vi "Netburner_cntl5.vi"() -> ()   [LabVIEW 2013]
uses:
  <vilib>/Analysis/NI_AALBase.lvlib
panel:
  out "Min ADC":dbl format="%#_5g"
  out "Max ADC":dbl format="%#_5g"
  out "ADC Voltage Chart":dbl(graph)
  out "# Cycles":i32
  out "ADC Std Dev":dbl format="%#_4g"
  out "Mean ADC":dbl format="%#_5g"
  out "ADC error":dbl[](array[numeric])
  out "ADC value":dbl[](array[numeric])
  out "#  Bytes Read End":u32
  out "End string":string
  out "ADC result string":string
  out "#  Bytes Read Data":u32
  in  "DAC, ADC String":string="0 1. 1 -1. 0 100 100"
  out "Error Out":errorcluster={"status"=FALSE, "code"=1073676294, "source"="VISA Read in Netburner_RD.vi->Netburner_cntl.vi"}
  in  "Error In (none)":errorcluster
  in  "COM Port #":refnum<visa-resource-name>="COM3"
  # "Netburner ADC/DAC Test Interface"
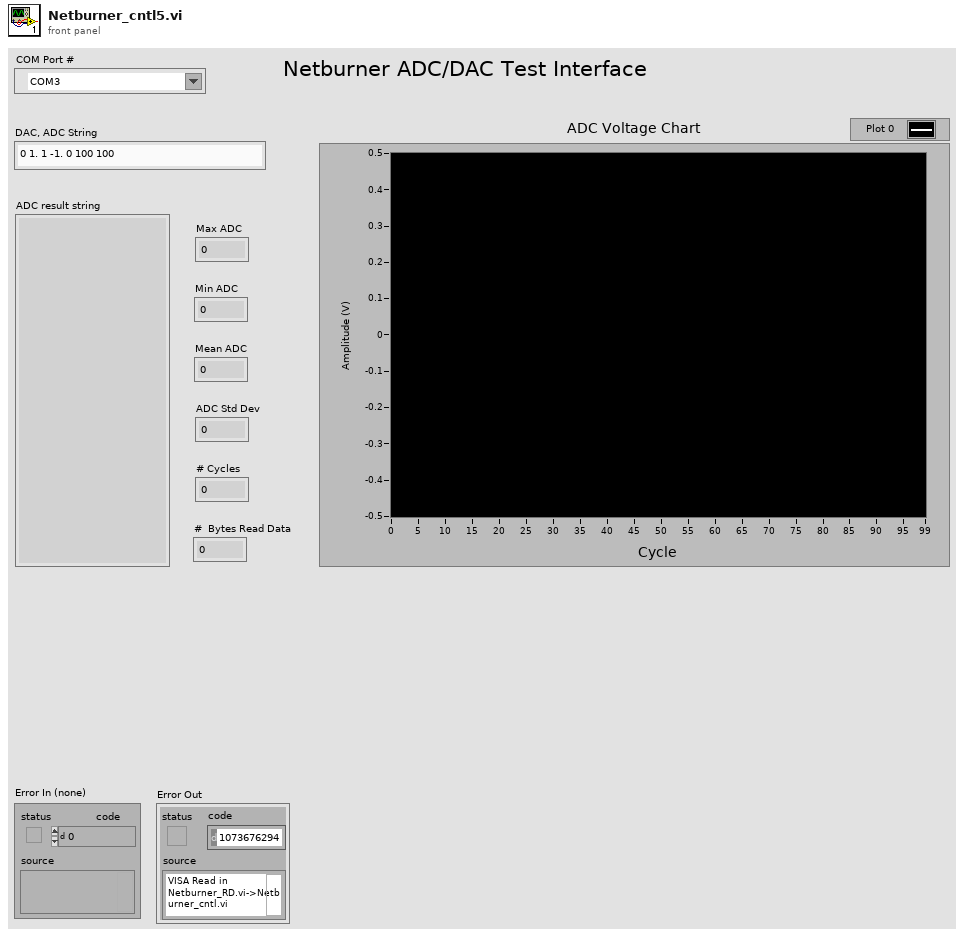
[diagram p1: front panel]
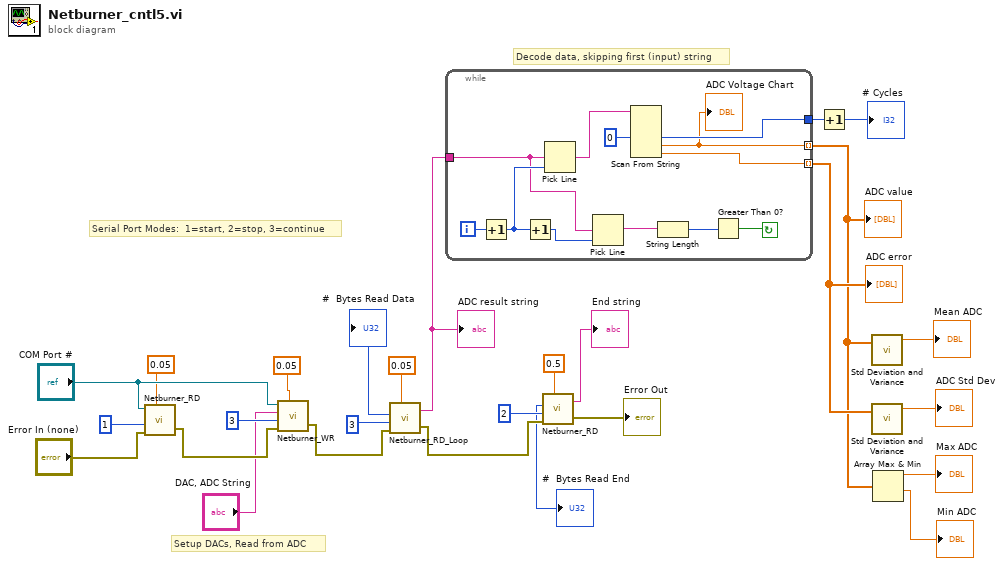
[diagram p0: block diagram]
diagram:
  # "Decode data, skipping first (input) string"
  # "Serial Port Modes:  1=start, 2=stop, 3=continue"
  # "Setup DACs, Read from ADC"
  n1 = call "Netburner_RD.vi"("VISA resource name (COM Port #)"="COM Port #", "Mode (0)"=1, "Error In (no error)"="Error In (none)", "Wait (sec)"=0.05) -> ("Error Out"=w26:errorcluster)  [unwired: 2 out]
  n2 = call "Netburner_WR.vi"("VISA resource name (COM Port #)"="COM Port #", "String to Send"="DAC, ADC String", "Mode (0)"=3, "Error In (no error)"=w26, "Wait (sec)"=0.05) -> ("Error Out"=w13:errorcluster)  [unwired: 1 in]
  n3 = call "Netburner_RD_Loop.vi"("Mode (0)"=3, "Error In (no error)"=w13, "Wait (sec)"=0.05) -> ("#  Bytes Read"=→"#  Bytes Read Data":u32, "Return String from Device"=w9:string, "Error Out"=w22:errorcluster)  [unwired: 1 in]
  "ADC result string" <- w9
  n4 = while {
    tunnel: w9 -> [w30]
    tunnel: [w34] -> w5
    tunnel: [w28] -> w3 mode=indexing
    tunnel: [w33] -> w8 mode=indexing
    i -> [w39]
    stop <- w35 continue-if-true
    n5 = Increment(x=w39) -> (x+1=w32:i32)
    n6 = Increment(x=w32) -> (x+1=w31:i32)
    n7 = Pick Line(multi-line string=w30, line index=w32) -> (output string=w37:string)  [unwired: 1 in]
    n8 = Pick Line(multi-line string=w30, line index=w31) -> (output string=w29:string)  [unwired: 1 in]
    n9 = Scan From String "Scan From String"(input string=w37, default 1=0) -> (output 1=w34:i32, output 2=w28:dbl, output 3=w33:dbl)  [unwired: 5 in, 3 out]
    "ADC Voltage Chart" <- w28
    n10 = String Length(string=w29) -> (length=w36:i32)
    n11 = Greater Than 0?(x=w36) -> (x > 0?=w35:bool)
  }
  "ADC value" <- w3
  "ADC error" <- w8
  n12 = call "Netburner_RD.vi"("Mode (0)"=2, "Error In (no error)"=w22, "Wait (sec)"=0.5) -> ("Number of Bytes Received"=→"#  Bytes Read End":u32, "Return String from Device"=→"End string":string, "Error Out"=→"Error Out":errorcluster)  [unwired: 1 in]
  n13 = Increment(x=w5) -> (x+1=→"# Cycles":i32)
  n14 = call <vilib>:"Std Deviation and Variance.vi"("X"=w3) -> ("mean"=→"Mean ADC":dbl)  [unwired: 1 in, 2 out]
  n15 = call <vilib>:"Std Deviation and Variance.vi"("X"=w8) -> ("mean"=→"ADC Std Dev":dbl)  [unwired: 1 in, 2 out]
  n16 = Array Max & Min(array=w3) -> (max value=→"Max ADC":dbl, min value=→"Min ADC":dbl)  [unwired: 2 out]
